vi "cRIO_4DoF_Fsample.vi"(11 "Sensor V offset":dbl[](array[numeric])) -> (2 "F":dbl[](array[numeric]), 3 "Array":dbl[](array[numeric]))   [LabVIEW 2019]
uses:
  <vilib>/imath/engines/lvmath2/RunTimeEngine/ArithmeticOperatorToken/NIMS_ArithmeticOperator_multmx(M,CV).vi
  <instcachedir>/0/NIMS_ArithmeticOperator_multmx(M,CV)_1D61EED49E1847F3B05DBB8EDD2FBF8F.lvgen/NIMS_ArithmeticOperator_multmx(M,CV)_1D61EED49E1847F3B05DBB8EDD2FBF8F_000.vi
  <vilib>/imathl/engines/lvmath/Functions/Error Handling/Create Error.vi
  <vilib>/imath/engines/lvmath2/RunTimeEngine/IndexRead/NIMS M(S,S).vi
  <instcachedir>/0/NIMS M(S,S)_AC51E74150A542F7991B9634C66F3096.lvgen/NIMS M(S,S)_AC51E74150A542F7991B9634C66F3096_000.vi
  <vilib>/imath/engines/lvmath2/RunTimeEngine/IndexReplace/NIMS M(S,S)=S.vi
  <instcachedir>/0/NIMS M(S,S)=S_F60428D0350A4667AE68E0C0372F4DD1.lvgen/NIMS M(S,S)=S_F60428D0350A4667AE68E0C0372F4DD1_000.vi
  <vilib>/imath/engines/lvmath2/RunTimeEngine/ErrorHandling/NIMS_Create Error From Enums.vi
  <vilib>/imath/engines/lvmath2/RunTimeEngine/NodeEndStatement/NIMS_NodeEndStatement_Output.vi
  <instcachedir>/0/NIMS_NodeEndStatement_Output_53EC0D466D134D7ABD903AC30B43404B.lvgen/NIMS_NodeEndStatement_Output_53EC0D466D134D7ABD903AC30B43404B_002.vi
  <vilib>/imath/engines/lvmath2/RunTimeEngine/ErrorHandling/NIMS_Finalize Error.vi
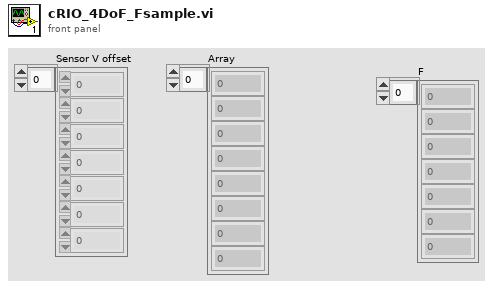
[diagram p1: front panel]
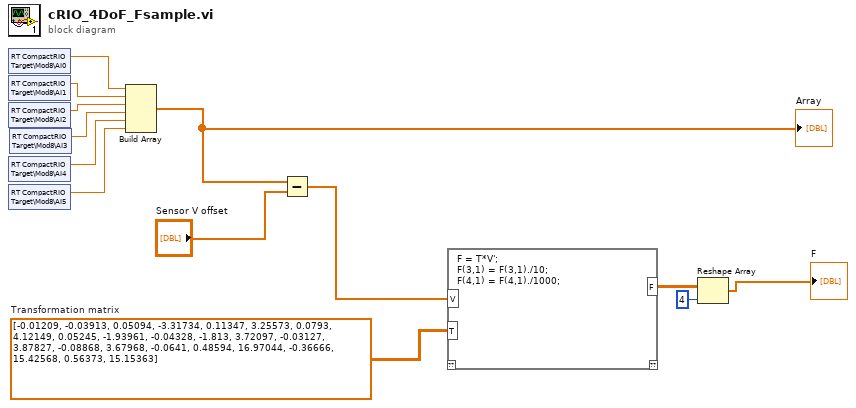
[diagram p0: block diagram]
diagram:
  w6 = dbl[][] [[-0.01209, -0.03913, 0.05094, -3.31734, 0.11347, 3.25573], [0.0793, 4.12149, 0.05245, -1.93961, -0.04328, -1.813], [3.72097, -0.03127, 3.87827, -0.08868, 3.67968, -0.0641], [0.48594, 16.97044, -0.36666, 15.42568, 0.56373, 15.15363]]  # Transformation matrix
  n1 = shared-variable "RT CompactRIO Target\\Mod8\\AI0"() -> (w3:dbl)  [unwired: 1 in, 1 out]
  n2 = shared-variable "RT CompactRIO Target\\Mod8\\AI1"() -> (w2:dbl)  [unwired: 1 in, 1 out]
  n3 = shared-variable "RT CompactRIO Target\\Mod8\\AI2"() -> (w1:dbl)  [unwired: 1 in, 1 out]
  n4 = shared-variable "RT CompactRIO Target\\Mod8\\AI4"() -> (w10:dbl)  [unwired: 1 in, 1 out]
  n5 = shared-variable "RT CompactRIO Target\\Mod8\\AI5"() -> (w11:dbl)  [unwired: 1 in, 1 out]
  n6 = shared-variable "RT CompactRIO Target\\Mod8\\AI3"() -> (w9:dbl)  [unwired: 1 in, 1 out]
  n7 = Build Array(w3, w2, w1, w9, w10, w11) -> (w12:dbl[])
  "Array" <- w12
  n8 = Subtract(x=w12, y="Sensor V offset") -> (x-y=w5:dbl[])
  n9 = mathscript code="F = T*V';\nF(3,1) = F(3,1)./10;\nF(4,1) = F(4,1)./1000;"("V"=w5, "T"=w6) -> ("F"=w7:dbl[][])  [unwired: 1 in, 1 out]
  n10 = Reshape Array(w7, 4 ("dimension size")) -> (→"F":dbl[])
